vi "Calibrate_power.vi"(8 "error in":errorcluster, 10 "Calibrate?":T1, 11 "FPGA VI Reference IN":refnum<k20>) -> (0 "error out":errorcluster, 1 "best fit":dynamicdata(graph), 2 "Fit Parameters":dbl[](array[numeric]), 3 "Power Values":dbl[](array[numeric]), 5 "AOM Volts":dbl[](array[numeric]))   [LabVIEW 2016]
uses:
  Calibrate_control.ctl
  Calibrate_enum.ctl
  <vilib>/Utility/error.llb/Error Cluster From Error Code.vi
  <vilib>/rvi/errors/niLvFpgaAdjustHostInterfaceError.vi
  <vilib>/Utility/file.llb/Write Delimited Spreadsheet (DBL).vi
  <vilib>/Utility/file.llb/Read Delimited Spreadsheet (DBL).vi
  <vilib>/rvi/interface/nirviReadWriteControl/nirviReadWriteControl.xnode
  NiFpgaLv.dll
  <vilib>/rvi/interface/Simulation/niFpgaSimulationCallBeginRW.vi
panel:
  out "Input needed":bool
  in  "YYMMDD of last calibration":string
  in  "OK":bool
  in  "Power (mW)":dbl
  # "If doing full calibration:"
  # "If doing Recall:"
  # "Hit ok button after you finish inputting data"
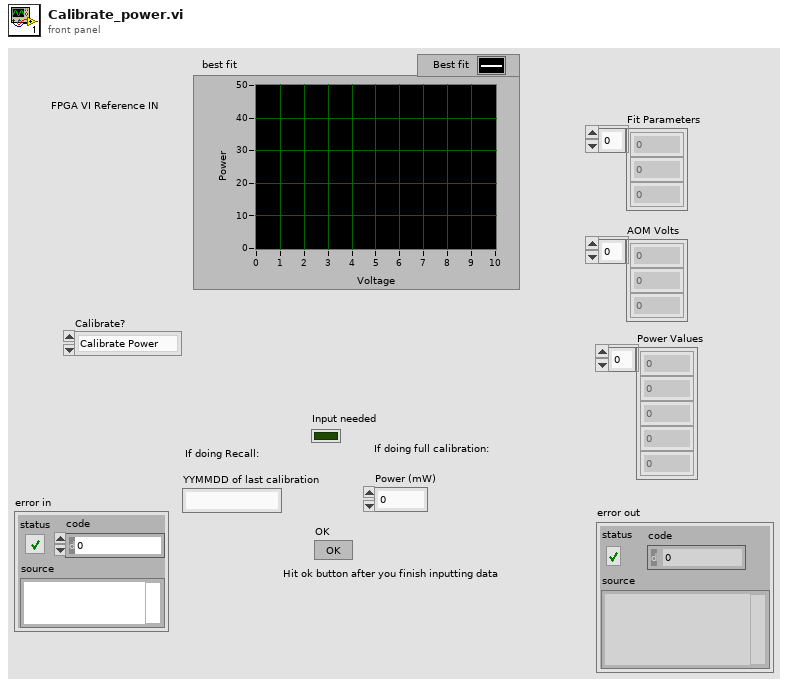
[diagram p1: front panel]
types:
  T1 = typedef "Calibrate_control.ctl" = enum16{"Calibrate Power", "Recall Calibration", "Use Voltage Only"}
  T2 = typedef "Calibrate_enum.ctl" = enum16{"Start", "Recall", "Measure", "Close", "Fit", "Save"}
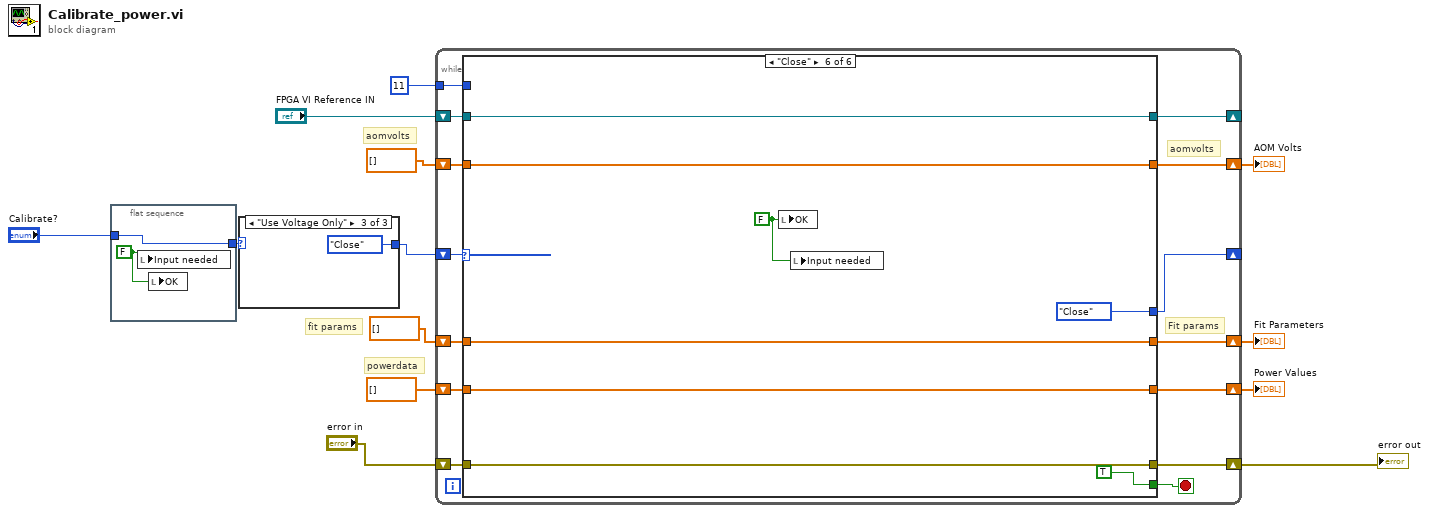
[diagram p0: block diagram]
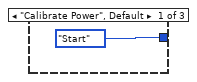
[diagram p2: hidden frame]
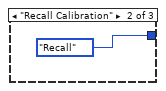
[diagram p3: hidden frame]
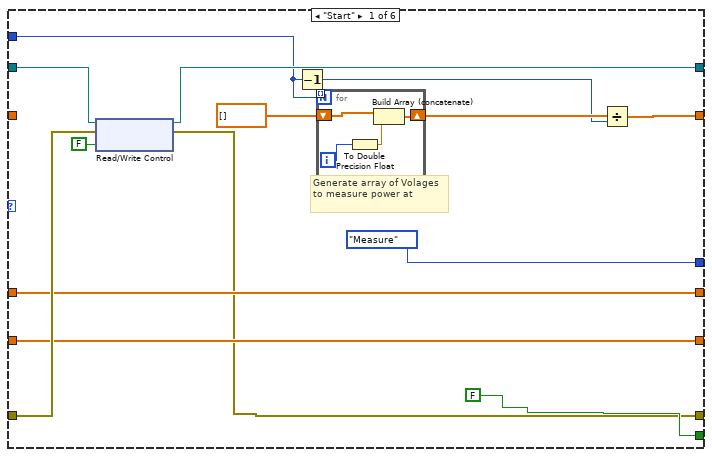
[diagram p4: hidden frame]
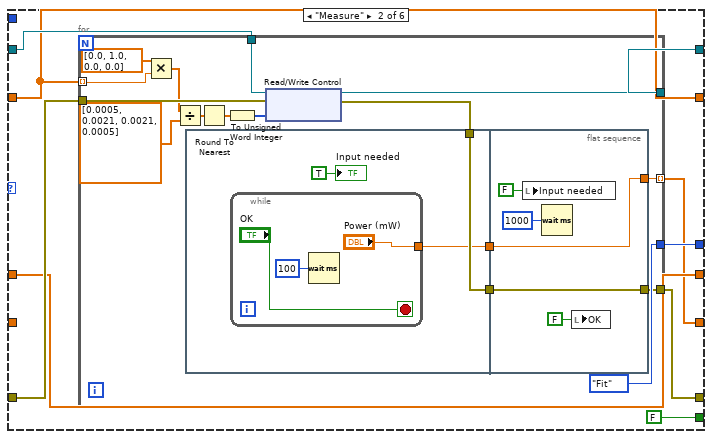
[diagram p5: hidden frame]
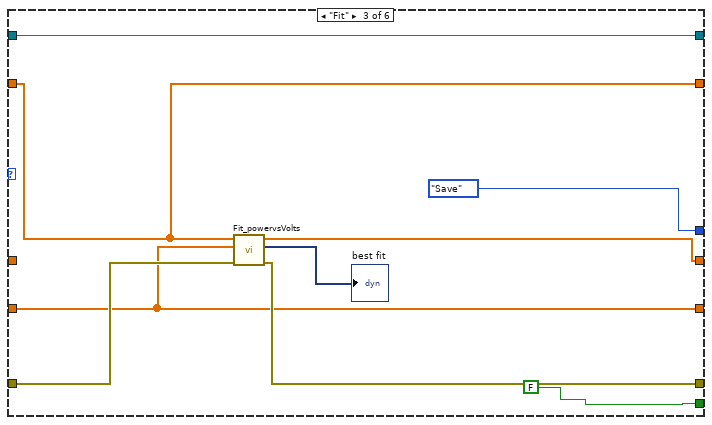
[diagram p6: hidden frame]
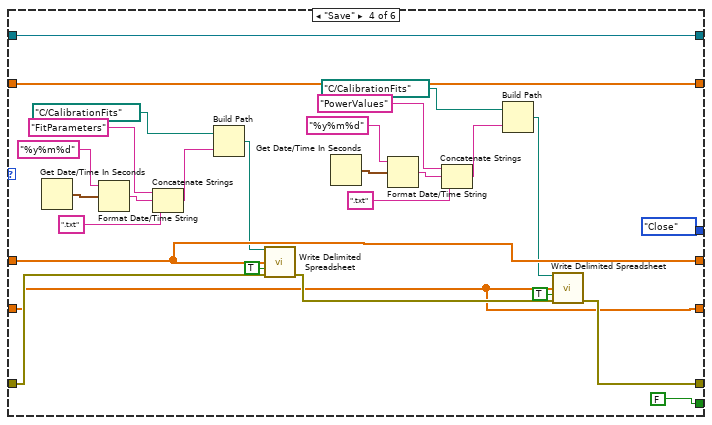
[diagram p7: hidden frame]
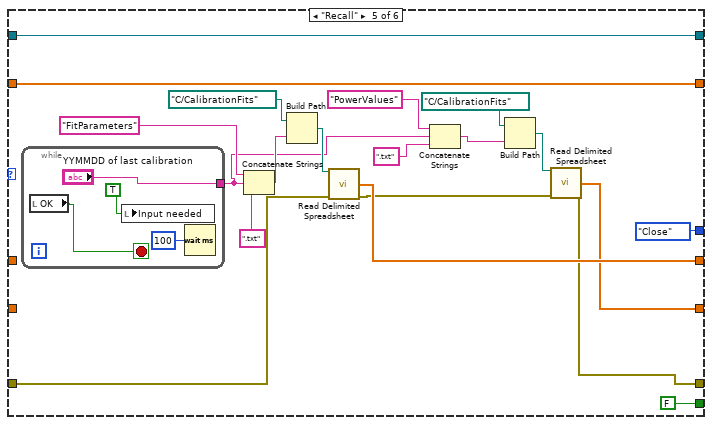
[diagram p8: hidden frame]
diagram:
  # "fit params"
  # "powerdata"
  # "aomvolts"
  n1 = flat-sequence {
    tunnel: "Calibrate?" -> [w15]
    tunnel: [w15] -> w7
    frame #0 {
      w14 = FALSE ("Measure Power now")
      n2 = local write "Input needed"(w14) -> ()
      n3 = local write "OK"(w14) -> ()
    }
  }
  n4 = case shown="\"Use Voltage Only\"" w7 {
    tunnel: [Calibrate_enum."Start" Calibrate_enum."Recall" Calibrate_enum."Close"] -> w8
    frame "Calibrate Power", Default {
    }
    frame "Recall Calibration" {
    }
    frame "Use Voltage Only" {
    }
  }
  n5 = while {
    shift-right: [w28] -> w4
    shift-left: "error in" -> [w31]
    shift-right: [w29] -> _
    shift-left: "FPGA VI Reference IN" -> [w30]
    shift-right: [w24] -> _
    shift-left: w8 -> [w32]
    shift-right: [w27] -> w3
    shift-left: dbl[] [] -> [w26]
    tunnel: 11 ("Cal. Num Pts") -> [w25]
    shift-right: [w23] -> w2
    shift-left: dbl[] [] -> [w22]
    shift-right: [w21] -> w9
    shift-left: dbl[] [] ("x_out") -> [w19]
    stop <- w20 stop-if-true
    # "aomvolts"
    # "Fit params"
    n6 = case shown="\"Close\"" w32 {
      tunnel: w31 -> [w46 w60 w96 w123 w134 w149]
      tunnel: w30 -> [w45 w59 w89 w117 w143 w153]
      tunnel: [w44 w58 w89 w117 w143 w153] -> w29
      tunnel: [w33 w53 w95 w99 w124 w149] -> w28
      tunnel: [w40 w56 w90 w119 w142 w152] -> w27
      tunnel: w26 -> [_ w56 w90 w119 w142 w152]
      tunnel: w25 -> [w38 _ _ _ _ _]
      tunnel: [Calibrate_enum."Measure" w57 Calibrate_enum."Save" Calibrate_enum."Close" Calibrate_enum."Close" Calibrate_enum."Close"] -> w24
      tunnel: [w36 w52 w93 w97 w125 w150] -> w23
      tunnel: w22 -> [w36 _ w93 w97 _ w150]
      tunnel: [w34 w54 w94 w120 w133 w151] -> w21
      tunnel: [FALSE FALSE FALSE FALSE FALSE TRUE] -> w20
      tunnel: w19 -> [w34 w54 _ w120 _ w151]
      frame "Start" {
        # "Generate array of Volages to measure power at"
        n7 = xnode "Read/Write Control"("FPGA VI Reference In"=w45, "error in"=w46, "Dymin On?"=FALSE) -> ("FPGA VI Reference Out"=w44:refnum<k20>, "error out"=w33:errorcluster)
        n8 = Decrement(x=w38) -> (x-1=w39:i32)
        n9 = for {
          N: w38 -> [w47]
          shift-right: [w50] -> w41
          shift-left: dbl[] [] -> [w51]
          tunnel: [w47] -> _ mode=indexing
          i -> [w49]
          n10 = To Double Precision Float(number=w49) -> (double precision float=w48:dbl)
          n11 = Build Array (concatenate)(w51, w48) -> (w50:dbl[])
        }
        n12 = Divide(x=w41, y=w39) -> (x/y=w40:dbl[])
      }
      frame "Measure" {
        n13 = for {
          tunnel: w60 -> [w72]
          tunnel: w56 -> [w70] mode=indexing
          tunnel: w59 -> [w68]
          tunnel: [w67] -> w58
          tunnel: [Calibrate_enum."Fit"] -> w57
          tunnel: [w63] -> w53
          tunnel: [w62] -> w52 mode=indexing
          n14 = Multiply(x=dbl[] [0.0, 1.0, 0.0, 0.0] ("Calibration Voltages"), y=w70) -> (x*y=w69:dbl[])
          n15 = Divide(x=w69, y=dbl[] [0.0005, 0.0021, 0.0021, 0.0005]) -> (x/y=w75:dbl[])
          n16 = flat-sequence {
            tunnel: w66 -> [w79]
            tunnel: [w79] -> w64
            tunnel: [w78] -> w61
            tunnel: [w86] -> w62
            tunnel: w64 -> [w87]
            tunnel: [w87] -> w63
            tunnel: w61 -> [w86]
            frame #0 {
              n17 = while {
                tunnel: ["Power (mW)"] -> w78
                stop <- "OK" stop-if-true
                n18 = Wait (ms)(milliseconds to wait=u32 100) -> ()  [unwired: 1 out]
              }
              "Input needed" <- TRUE ("Input needed")
            }
            frame #1 {
              n19 = local write "Input needed"(FALSE ("Input needed")) -> ()
              n20 = Wait (ms)(milliseconds to wait=u32 1000) -> ()  [unwired: 1 out]
              n21 = local write "OK"(FALSE ("OK")) -> ()
            }
          }
          n22 = Round To Nearest(number=w75) -> (nearest integer value=w74:dbl[])
          n23 = To Unsigned Word Integer(number=w74) -> (unsigned 16bit integer=w73:u16[])
          n24 = xnode "Read/Write Control"("FPGA VI Reference In"=w68, "error in"=w72, "AOM Volts"=w73) -> ("FPGA VI Reference Out"=w67:refnum<k20>, "error out"=w66:errorcluster)
        }
      }
      frame "Fit" {
        n25 = call "Fit_powervsVolts.vi"("error in"=w96, "powerdata"=w93, "aomdata"=w90) -> ("error out"=w95:errorcluster, "best fit"=→"best fit":dynamicdata, "x_out"=w94:dbl[])  [unwired: 6 in]
      }
      frame "Save" {
        n26 = Get Date/Time In Seconds() -> (seconds since 1Jan1904=w115:timestamp)
        n27 = Format Date/Time String(time format string (%c)="%y%m%d", seconds (now)=w115) -> (date/time string=w112:string)  [unwired: 1 in]
        n28 = Concatenate Strings("FitParameters", w112, ".txt" ("string")) -> (w110:string)
        n29 = Build Path(base path=path "C:/CalibrationFits", name or relative path=w110) -> (appended path=w109:path)
        n30 = call-poly <vilib>:"Write Delimited Spreadsheet.vi"("file path (dialog if empty)"=w109, "1D data"=w120, "append to file? (new file:F)"=TRUE, "error in (no error)"=w123) -> ("error out"=w100:errorcluster)  [unwired: 10 in, 1 out]
        n31 = Get Date/Time In Seconds() -> (seconds since 1Jan1904=w103:timestamp)
        n32 = Format Date/Time String(time format string (%c)="%y%m%d", seconds (now)=w103) -> (date/time string=w106:string)  [unwired: 1 in]
        n33 = Concatenate Strings("PowerValues", w106, ".txt" ("string")) -> (w108:string)
        n34 = Build Path(base path=path "C:/CalibrationFits", name or relative path=w108) -> (appended path=w98:path)
        n35 = call-poly <vilib>:"Write Delimited Spreadsheet.vi"("file path (dialog if empty)"=w98, "1D data"=w97, "append to file? (new file:F)"=TRUE, "error in (no error)"=w100) -> ("error out"=w99:errorcluster)  [unwired: 10 in, 1 out]
      }
      frame "Recall" {
        n36 = while {
          tunnel: ["YYMMDD of last calibration"] -> w131
          stop <- w145 stop-if-true
          n37 = local read "OK"() -> (w145:bool)
          n38 = local write "Input needed"(TRUE ("Input needed")) -> ()
          n39 = Wait (ms)(milliseconds to wait=u32 100) -> ()  [unwired: 1 out]
        }
        n40 = Concatenate Strings("FitParameters", w131, ".txt" ("string")) -> (w136:string)
        n41 = Build Path(base path=path "C:/CalibrationFits", name or relative path=w136) -> (appended path=w135:path)
        n42 = call-poly <vilib>:"Read Delimited Spreadsheet.vi"("file path (dialog if empty)"=w135, "error in (no error)"=w134) -> ("first row"=w133:dbl[], "error out"=w126:errorcluster)  [unwired: 8 in, 4 out]
        n43 = Concatenate Strings("PowerValues", w131, ".txt" ("string")) -> (w128:string)
        n44 = Build Path(base path=path "C:/CalibrationFits", name or relative path=w128) -> (appended path=w127:path)
        n45 = call-poly <vilib>:"Read Delimited Spreadsheet.vi"("file path (dialog if empty)"=w127, "error in (no error)"=w126) -> ("first row"=w125:dbl[], "error out"=w124:errorcluster)  [unwired: 8 in, 4 out]
      }
      frame "Close" {
        w154 = FALSE ("OK")
        n46 = local write "OK"(w154) -> ()
        n47 = local write "Input needed"(w154) -> ()
      }
    }
  }
  "error out" <- w4
  "Fit Parameters" <- w9
  "AOM Volts" <- w3
  "Power Values" <- w2
